vi "command.vi"(0 "HGF_GPG":refnum<class "HGF_GPG.lvclass">, 1 "options file":path, 2 "keyringfile":path, 3 "Sec keyringfile":path, 4 "targetfile":path, 5 "sourcefile":path, 7 "error in (no error)":errorcluster, 8 "key-id":string, 9 "overwrite? (t)":bool=TRUE, 10 "Trust DB":path, 11 "reveiver":string[](array[string]), 12 "task":T1(ring), 13 "password":string) -> (15 "standard output":string, 16 "dup Trust DB":path, 17 "data error":bool, 19 "return code":i32, 20 "dup HGF_GPG":refnum<class "HGF_GPG.lvclass">, 21 "dup options file":path, 22 "dup keyringfile":path, 23 "dup Sec keyringfile":path, 24 "dup targetfile":path, 25 "dup sourcefile":path, 26 "standard error":string, 27 "error out":errorcluster)   [LabVIEW 2012, in "HGF_GPG.lvlib" / "HGF_GPG.lvclass"]
doc: "VI executes following gpg-commands (commandline):\nEncrypt\nDecrypt\nSign\nVerify\nSign&Encrypt\nVerify&Decrypt"
uses:
  HGF_GPG.lvclass
  HGF_GPG.lvclass/HGF_GPG.ctl
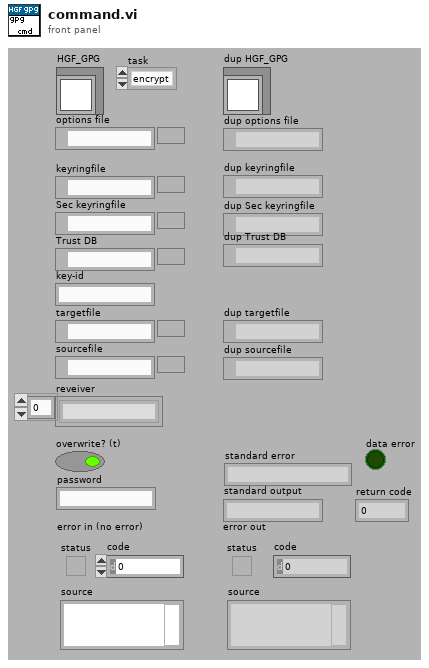
[diagram p1: front panel]
types:
  T1 = enum16{"encrypt", "decrypt", "sign", "verify", "sign & encrypt", "verify & decrypt"}
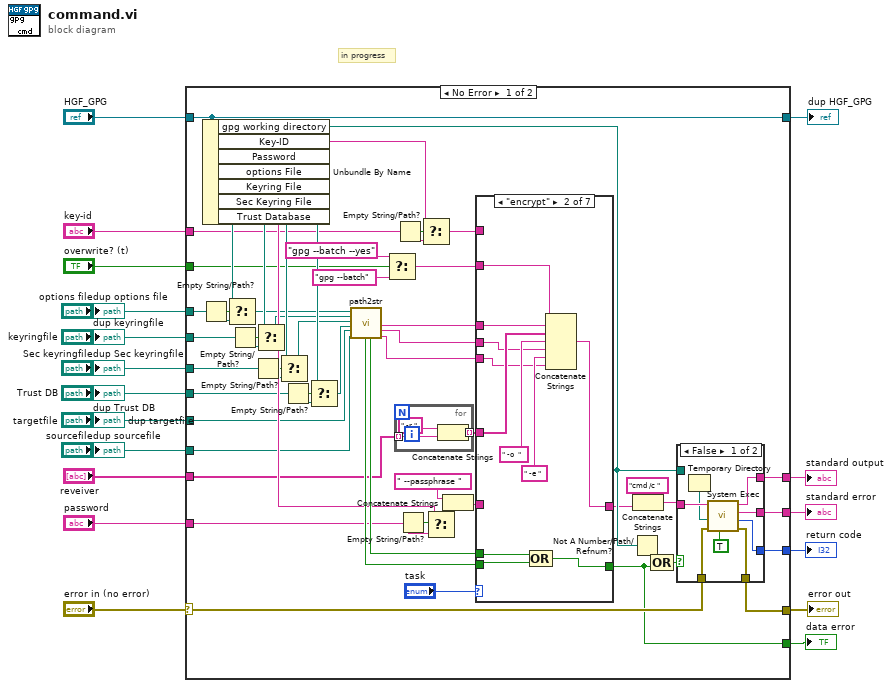
[diagram p0: block diagram]
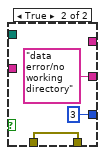
[diagram p2: hidden frame]
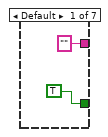
[diagram p3: hidden frame]
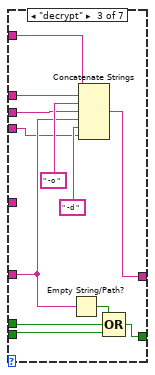
[diagram p4: hidden frame]
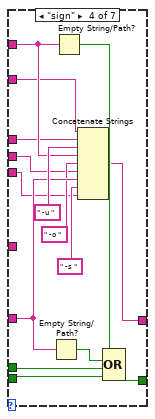
[diagram p5: hidden frame]
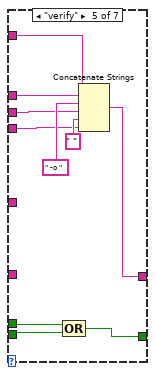
[diagram p6: hidden frame]
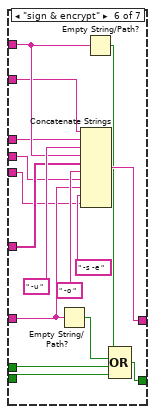
[diagram p7: hidden frame]
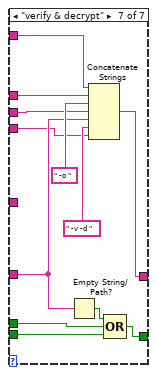
[diagram p8: hidden frame]
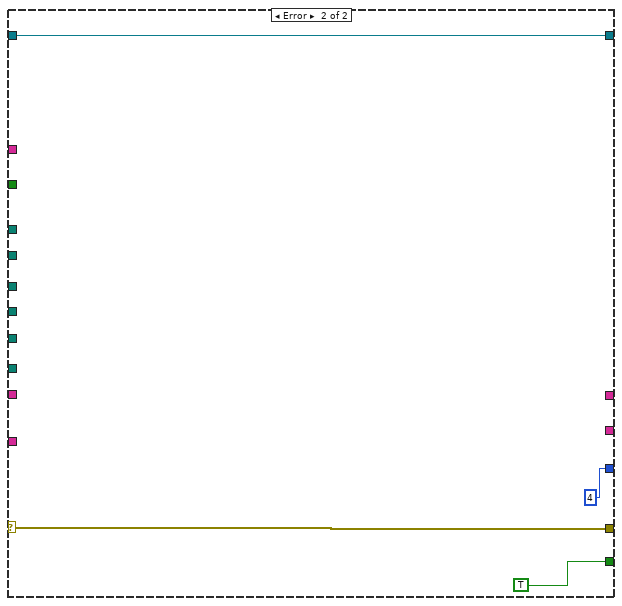
[diagram p9: hidden frame]
diagram:
  # "in progress"
  n1 = case shown="No Error" "error in (no error)" {
    selector: "error in (no error)" -> [w54 w167]
    tunnel: [w53 w167] -> w17
    tunnel: [w60 w166] -> w15
    tunnel: "HGF_GPG" -> [w60 w166]
    tunnel: "overwrite? (t)" -> [w62 _]
    tunnel: "reveiver" -> [w61 _]
    tunnel: "targetfile" -> [w32 _]
    tunnel: "password" -> [w58 _]
    tunnel: "sourcefile" -> [w33 _]
    tunnel: [w52 _] -> w11
    tunnel: [w51 _] -> w10
    tunnel: [w50 4 ("return code")] -> w9
    tunnel: [w44 TRUE] -> w8
    tunnel: "key-id" -> [w39 _]
    tunnel: "options file" -> [w30 _]
    tunnel: "keyringfile" -> [w27 _]
    tunnel: "Sec keyringfile" -> [w25 _]
    tunnel: "Trust DB" -> [w20 _]
    frame No Error {
      n2 = Empty String/Path?(string/path=w30) -> (empty?=w31:bool)
      n3 = Unbundle By Name(w60) -> ("gpg working directory"=w64:path, "Key-ID"=w42:string, "Password"=w67:string, "options File"=w66:path, "Keyring File"=w65:path, "Sec Keyring File"=w70:path, "Trust Database"=w71:path)
      n4 = Select(t=w66, s=w31, f=w30) -> (s? t:f=w29:path)
      n5 = Empty String/Path?(string/path=w27) -> (empty?=w28:bool)
      n6 = Empty String/Path?(string/path=w25) -> (empty?=w26:bool)
      n7 = Select(t=w65, s=w28, f=w27) -> (s? t:f=w23:path)
      n8 = Select(t=w70, s=w26, f=w25) -> (s? t:f=w22:path)
      n9 = Empty String/Path?(string/path=w20) -> (empty?=w21:bool)
      n10 = Select(t=w71, s=w21, f=w20) -> (s? t:f=w19:path)
      n11 = call "path2str.vi"("options file"=w29, "keyringfile"=w23, "Sec keyringfile"=w22, "Trust DB"=w19, "targetfile"=w32, "sourcefile"=w33) -> ("tf NaPath"=w69:bool, "sf NaPath"=w68:bool, "opt/keyr/seckeyr/trusdb"=w24:string, "targetfile path"=w35:string, "sourcefile path"=w34:string)  [unwired: 9 out]
      n12 = Select(t="gpg --batch --yes", s=w62, f="gpg --batch") -> (s? t:f=w56:string)
      n13 = Empty String/Path?(string/path=w39) -> (empty?=w40:bool)
      n14 = for {
        tunnel: w61 -> [w73] mode=indexing
        tunnel: [w72] -> w55 mode=indexing
        n15 = Concatenate Strings(" -r ", w73) -> (w72:string)
      }
      n16 = Empty String/Path?(string/path=w58) -> (empty?=w59:bool)
      n17 = Select(t=w42, s=w40, f=w39) -> (s? t:f=w41:string)
      n18 = Select(t=w67, s=w59, f=w58) -> (s? t:f=w49:string)
      n19 = Concatenate Strings(" --passphrase ", w49) -> (w48:string)
      n20 = case shown="\"encrypt\"" "task" {
        tunnel: w56 -> [_ w96 w108 w113 w133 w141 w160]
        tunnel: w55 -> [_ w95 _ _ _ w147 _]
        tunnel: w35 -> [_ w94 w107 w119 w132 w146 w159]
        tunnel: w34 -> [_ w93 w101 w118 w131 w136 w158]
        tunnel: w48 -> [_ _ w109 w124 _ w140 w161]
        tunnel: ["" w92 w106 w117 w130 w145 w157] -> w37
        tunnel: w68 -> [_ w90 w104 w115 w128 w143 w155]
        tunnel: w69 -> [_ w91 w105 w116 w129 w144 w156]
        tunnel: [TRUE w89 w103 w114 w127 w142 w154] -> w44
        tunnel: w41 -> [_ _ _ w120 _ w148 _]
        tunnel: w24 -> [_ w88 w99 w111 w126 w137 w152]
        frame Default {
        }
        frame "encrypt" {
          n21 = Compound Arithmetic op=OR(w91, w90) -> (w89:bool)
          n22 = Concatenate Strings(w96, w88, w95, " -o  " ("string"), w94, " -e " ("string"), w93) -> (w92:string)
        }
        frame "decrypt" {
          n23 = Empty String/Path?(string/path=w109) -> (empty?=w100:bool)
          n24 = Concatenate Strings(w108, w99, " -o ", w107, w109, " -d " ("string"), w101) -> (w106:string)
          n25 = Compound Arithmetic op=OR(w100, w105, w104) -> (w103:bool)
        }
        frame "sign" {
          n26 = Empty String/Path?(string/path=w124) -> (empty?=w112:bool)
          n27 = Empty String/Path?(string/path=w120) -> (empty?=w121:bool)
          n28 = Concatenate Strings(w113, w111, " -u " ("use key id"), w120, " -o " ("output file"), w119, w124, " -s " ("sign file"), w118) -> (w117:string)
          n29 = Compound Arithmetic op=OR(w121, w112, w116, w115) -> (w114:bool)
        }
        frame "verify" {
          n30 = Compound Arithmetic op=OR(w129, w128) -> (w127:bool)
          n31 = Concatenate Strings(w133, w126, " -o " ("string"), w132, " " ("string"), w131) -> (w130:string)
        }
        frame "sign & encrypt" {
          n32 = Empty String/Path?(string/path=w140) -> (empty?=w139:bool)
          n33 = Concatenate Strings(w141, w137, " -u " ("use Key-ID"), w148, w147, " -o " ("output file"), w146, w140, " -s -e " ("sign & encrypt file"), w136) -> (w145:string)
          n34 = Empty String/Path?(string/path=w148) -> (empty?=w138:bool)
          n35 = Compound Arithmetic op=OR(w138, w139, w144, w143) -> (w142:bool)
        }
        frame "verify & decrypt" {
          n36 = Empty String/Path?(string/path=w161) -> (empty?=w153:bool)
          n37 = Concatenate Strings(w160, w152, " -o " ("output file"), w159, w161, " -v -d " ("verify and decrypt"), w158) -> (w157:string)
          n38 = Compound Arithmetic op=OR(w153, w156, w155) -> (w154:bool)
        }
      }
      n39 = Not A Number/Path/Refnum?(number/path/refnum=w64) -> (NaN/Path/Refnum?=w46:bool)
      n40 = Concatenate Strings("cmd /c " ("string"), w37) -> (w36:string)
      n41 = Compound Arithmetic op=OR(w46, w44) -> (w45:bool)
      n42 = case shown="False" w45 {
        tunnel: w54 -> [w81 w85]
        tunnel: [w80 w85] -> w53
        tunnel: w64 -> [_ _]
        tunnel: w36 -> [w79 _]
        tunnel: [w78 _] -> w52
        tunnel: [w77 "data error/no working directory" ("standard error")] -> w51
        tunnel: [w76 3 ("return code")] -> w50
        frame False {
          n43 = Temporary Directory() -> (w75:path)
          n44 = call <vilib>:"System Exec.vi"("run minimized? (F)"=TRUE, "error in (no error)"=w81, "working directory"=w75, "command line"=w79) -> ("error out"=w80:errorcluster, "return code"=w76:i32, "standard error"=w77:string, "standard output"=w78:string)  [unwired: 2 in, 2 out]
        }
        frame True {
        }
      }
    }
    frame Error {
    }
  }
  "error out" <- w17
  "dup HGF_GPG" <- w15
  "standard output" <- w11
  "standard error" <- w10
  "return code" <- w9
  "data error" <- w8
  "dup targetfile" <- "targetfile"
  "dup sourcefile" <- "sourcefile"
  "dup options file" <- "options file"
  "dup keyringfile" <- "keyringfile"
  "dup Sec keyringfile" <- "Sec keyringfile"
  "dup Trust DB" <- "Trust DB"
